vi "uTTA_Write_UCF_File.vi"(4 "TC_Channels":T1(array[cluster]), 6 "TSP_Channels":T1(array[cluster]), 8 "error in (no error)":errorcluster, 10 "Inputs":T2 {"I_Sense Offset" format="%#3.3pA"; "I_Sense Gain" format="%#3.3pA/Digit"; "CH_I Offset" format="%#3.3pA"; "CH_I Gain" format="%#3.3pA/Digit"; "CH0 PA3 Offset" format="%#3.3pV"; "CH0 PA3 Gain" format="%#3.3pV/Digit"; "CH0 PA2 Offset" format="%#3.3pV"; "CH0 PA2 Gain" format="%#3.3pV/Digit"; "CH0 PA1 Offset" format="%#3.3pV"; "CH0 PA1 Gain" format="%#3.3pV/Digit"; "CH0 PA0 Offset" format="%#3.3pV"; "CH0 PA0 Gain" format="%#3.3pV/Digit"; "CH3 PA0 Offset" format="%#3.3pV"; "CH3 PA0 Gain" format="%#3.3pV/Digit"; "CH2 PA0 Offset" format="%#3.3pV"; "CH2 PA0 Gain" format="%#3.3pV/Digit"; "CH1 PA0 Offset" format="%#3.3pV"; "CH1 PA0 Gain" format="%#3.3pV/Digit"; "Voffs1 Offset" format="%#3.3pV"; "Voffs1 Gain" format="%#3.3pV/Digit"; "Voffs0 Offset" format="%#3.3pV"; "CH3 Diff Gain" format="%#3.3pV/V"; "CH2 Diff Gain" format="%#3.3pV/V"; "CH1 Diff Gain" format="%#3.3pV/V"; "Voffs0 Gain" format="%#3.3pV/Digit"; "CH0 Diff Gain" format="%#3.3pV/V"}, 11 "selected path":path) -> (0 "error out":errorcluster, 3 "file path":path)   [LabVIEW 2021]
uses:
  CTL_uTTA_BlockDiagCal.ctl
  <vilib>/Utility/config.llb/NI_LVConfig.lvlib
panel:
  # "G0"
  # "G1"
  # "G2"
  # "G3"
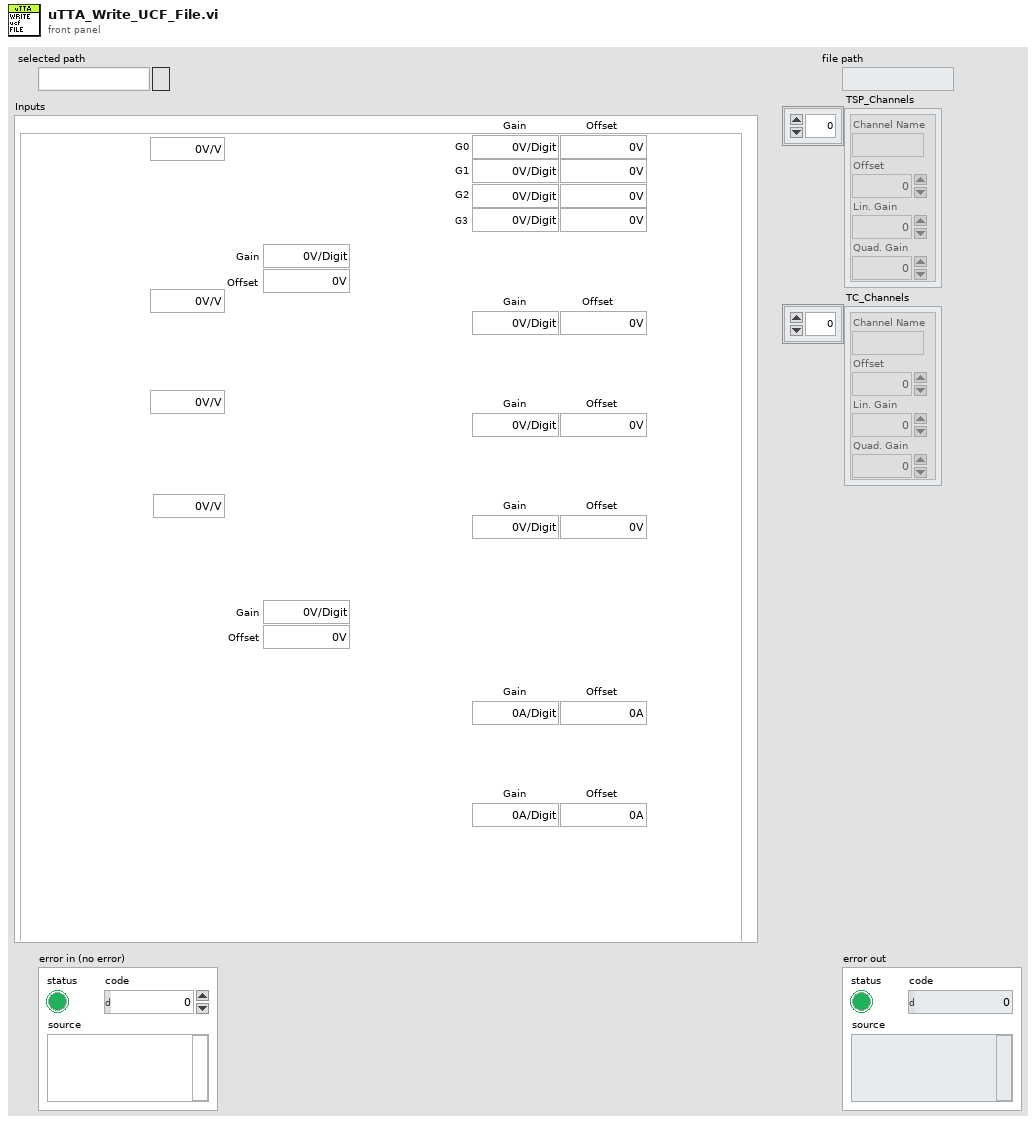
[diagram p1: front panel]
types:
  T1 = cluster{"Channel Name":string, "Offset":dbl, "Lin. Gain":dbl, "Quad. Gain":dbl}[]
  T2 = typedef "CTL_uTTA_BlockDiagCal.ctl" = cluster{"CH0 Diff Gain":dbl, "Voffs0 Gain":dbl, "CH1 Diff Gain":dbl, "CH2 Diff Gain":dbl, "CH3 Diff Gain":dbl, "Voffs0 Offset":dbl, "Voffs1 Gain":dbl, "Voffs1 Offset":dbl, "CH1 PA0 Gain":dbl, "CH1 PA0 Offset":dbl, "CH2 PA0 Gain":dbl, "CH2 PA0 Offset":dbl, "CH3 PA0 Gain":dbl, "CH3 PA0 Offset":dbl, "CH0 PA0 Gain":dbl, "CH0 PA0 Offset":dbl, "CH0 PA1 Gain":dbl, "CH0 PA1 Offset":dbl, "CH0 PA2 Gain":dbl, "CH0 PA2 Offset":dbl, "CH0 PA3 Gain":dbl, "CH0 PA3 Offset":dbl, "CH_I Gain":dbl, "CH_I Offset":dbl, "I_Sense Gain":dbl, "I_Sense Offset":dbl}
  T3 = typedef "NI_LVConfig.lvlib/Config Data RefNum.ctl" = refnum<k1>
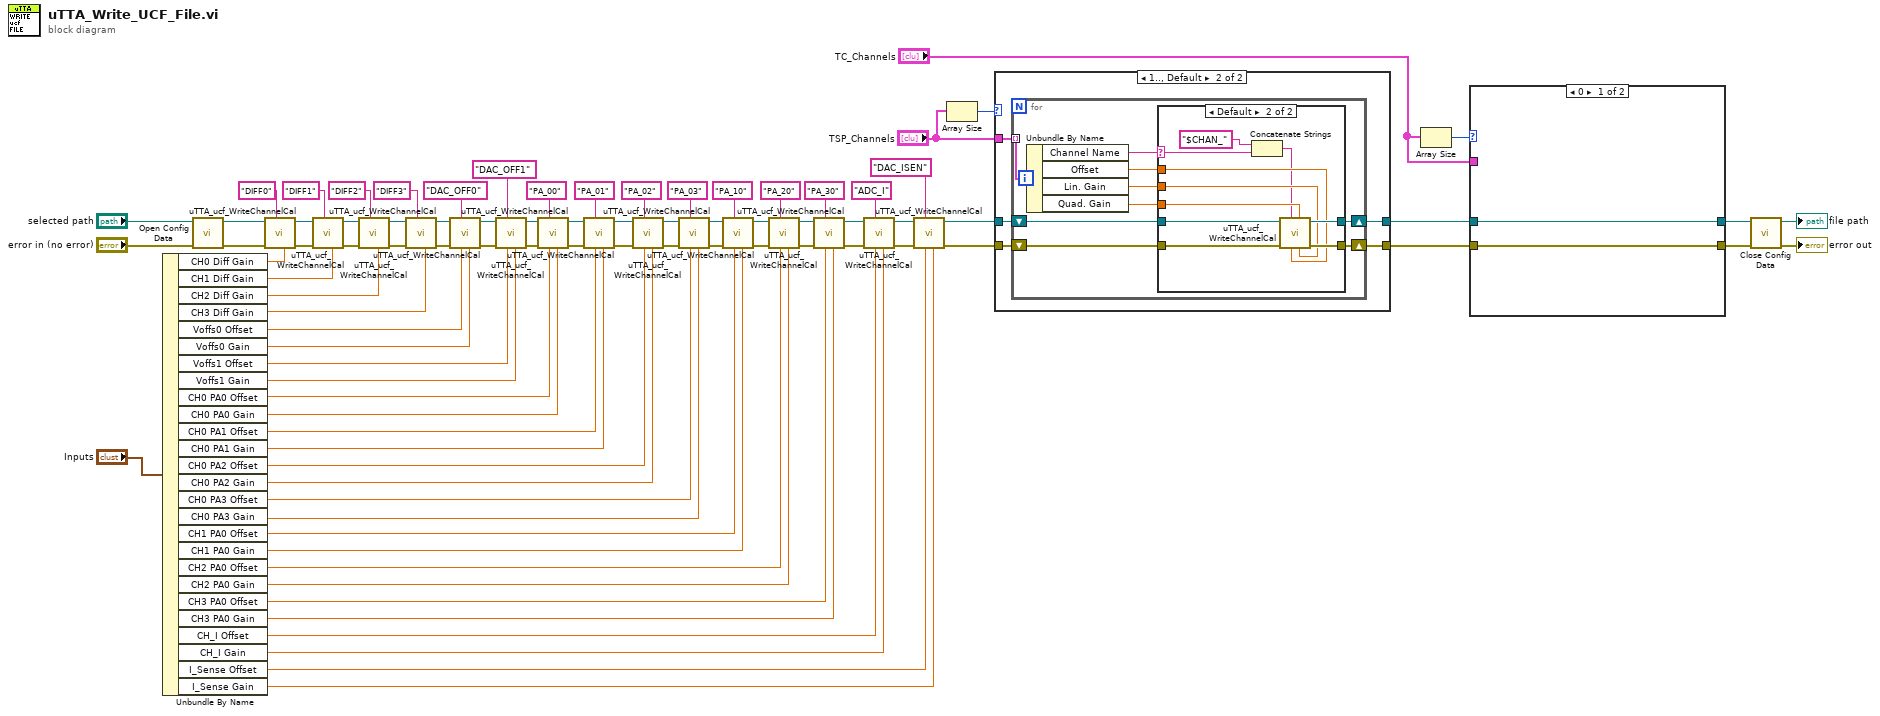
[diagram p0: block diagram]
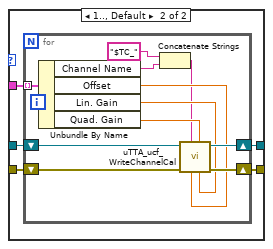
[diagram p2: hidden frame]
diagram:
  n1 = Unbundle By Name("Inputs") -> ("CH0 Diff Gain"=w28:dbl, "CH1 Diff Gain"=w29:dbl, "CH2 Diff Gain"=w30:dbl, "CH3 Diff Gain"=w33:dbl, "Voffs0 Offset"=w36:dbl, "Voffs0 Gain"=w37:dbl, "Voffs1 Offset"=w46:dbl, "Voffs1 Gain"=w47:dbl, "CH0 PA0 Offset"=w48:dbl, "CH0 PA0 Gain"=w49:dbl, "CH0 PA1 Offset"=w50:dbl, "CH0 PA1 Gain"=w51:dbl, "CH0 PA2 Offset"=w52:dbl, "CH0 PA2 Gain"=w53:dbl, "CH0 PA3 Offset"=w60:dbl, "CH0 PA3 Gain"=w61:dbl, "CH1 PA0 Offset"=w62:dbl, "CH1 PA0 Gain"=w63:dbl, "CH2 PA0 Offset"=w64:dbl, "CH2 PA0 Gain"=w65:dbl, "CH3 PA0 Offset"=w68:dbl, "CH3 PA0 Gain"=w69:dbl, "CH_I Offset"=w75:dbl, "CH_I Gain"=w76:dbl, "I_Sense Offset"=w15:dbl, "I_Sense Gain"=w14:dbl)
  n2 = call <vilib>:"Open Config Data.vi"("error in (no error)"="error in (no error)", "configuration file path"="selected path") -> ("error out"=w18:errorcluster, "refnum"=w19:T3)  [unwired: 7 in, 1 out]
  n3 = call "uTTA_ucf_WriteChannelCal.vi"("LinGain"=w28, "Section"="DIFF0" ("section"), "error in (no error)"=w18, "ucf FileRef in"=w19) -> ("error out"=w24:errorcluster, "ucf FileRef out"=w25:T3)  [unwired: 6 in]
  n4 = call "uTTA_ucf_WriteChannelCal.vi"("LinGain"=w29, "Section"="DIFF1" ("section"), "error in (no error)"=w24, "ucf FileRef in"=w25) -> ("error out"=w26:errorcluster, "ucf FileRef out"=w27:T3)  [unwired: 6 in]
  n5 = call "uTTA_ucf_WriteChannelCal.vi"("LinGain"=w30, "Section"="DIFF2" ("section"), "error in (no error)"=w26, "ucf FileRef in"=w27) -> ("error out"=w31:errorcluster, "ucf FileRef out"=w32:T3)  [unwired: 6 in]
  n6 = call "uTTA_ucf_WriteChannelCal.vi"("LinGain"=w33, "Section"="DIFF3" ("section"), "error in (no error)"=w31, "ucf FileRef in"=w32) -> ("error out"=w34:errorcluster, "ucf FileRef out"=w35:T3)  [unwired: 6 in]
  n7 = call "uTTA_ucf_WriteChannelCal.vi"("LinGain"=w37, "Offset"=w36, "Section"="DAC_OFF0", "error in (no error)"=w34, "ucf FileRef in"=w35) -> ("error out"=w38:errorcluster, "ucf FileRef out"=w39:T3)  [unwired: 5 in]
  n8 = call "uTTA_ucf_WriteChannelCal.vi"("LinGain"=w47, "Offset"=w46, "Section"="DAC_OFF1", "error in (no error)"=w38, "ucf FileRef in"=w39) -> ("error out"=w40:errorcluster, "ucf FileRef out"=w41:T3)  [unwired: 5 in]
  n9 = call "uTTA_ucf_WriteChannelCal.vi"("LinGain"=w49, "Offset"=w48, "Section"="PA_00", "error in (no error)"=w40, "ucf FileRef in"=w41) -> ("error out"=w42:errorcluster, "ucf FileRef out"=w43:T3)  [unwired: 5 in]
  n10 = call "uTTA_ucf_WriteChannelCal.vi"("LinGain"=w51, "Offset"=w50, "Section"="PA_01", "error in (no error)"=w42, "ucf FileRef in"=w43) -> ("error out"=w44:errorcluster, "ucf FileRef out"=w45:T3)  [unwired: 5 in]
  n11 = call "uTTA_ucf_WriteChannelCal.vi"("LinGain"=w53, "Offset"=w52, "Section"="PA_02", "error in (no error)"=w44, "ucf FileRef in"=w45) -> ("error out"=w54:errorcluster, "ucf FileRef out"=w55:T3)  [unwired: 5 in]
  n12 = call "uTTA_ucf_WriteChannelCal.vi"("LinGain"=w61, "Offset"=w60, "Section"="PA_03", "error in (no error)"=w54, "ucf FileRef in"=w55) -> ("error out"=w56:errorcluster, "ucf FileRef out"=w57:T3)  [unwired: 5 in]
  n13 = call "uTTA_ucf_WriteChannelCal.vi"("LinGain"=w63, "Offset"=w62, "Section"="PA_10", "error in (no error)"=w56, "ucf FileRef in"=w57) -> ("error out"=w58:errorcluster, "ucf FileRef out"=w59:T3)  [unwired: 5 in]
  n14 = call "uTTA_ucf_WriteChannelCal.vi"("LinGain"=w65, "Offset"=w64, "Section"="PA_20", "error in (no error)"=w58, "ucf FileRef in"=w59) -> ("error out"=w66:errorcluster, "ucf FileRef out"=w67:T3)  [unwired: 5 in]
  n15 = call "uTTA_ucf_WriteChannelCal.vi"("LinGain"=w69, "Offset"=w68, "Section"="PA_30", "error in (no error)"=w66, "ucf FileRef in"=w67) -> ("error out"=w73:errorcluster, "ucf FileRef out"=w74:T3)  [unwired: 5 in]
  n16 = call "uTTA_ucf_WriteChannelCal.vi"("LinGain"=w76, "Offset"=w75, "Section"="ADC_I", "error in (no error)"=w73, "ucf FileRef in"=w74) -> ("error out"=w17:errorcluster, "ucf FileRef out"=w16:T3)  [unwired: 5 in]
  n17 = call "uTTA_ucf_WriteChannelCal.vi"("LinGain"=w14, "Offset"=w15, "Section"="DAC_ISEN", "error in (no error)"=w17, "ucf FileRef in"=w16) -> ("error out"=w11:errorcluster, "ucf FileRef out"=w12:T3)  [unwired: 5 in]
  n18 = Array Size(array="TSP_Channels") -> (size(s)=w3:i32)
  n19 = case shown="1.., Default" w3 {
    tunnel: w12 -> [w88 w93]
    tunnel: w11 -> [w87 w92]
    tunnel: [w88 w91] -> w8
    tunnel: [w87 w90] -> w7
    tunnel: "TSP_Channels" -> [_ w89]
    frame 0 {
    }
    frame 1.., Default {
      n20 = for {
        shift-right: [w99] -> w91
        shift-left: w93 -> [w101]
        shift-right: [w98] -> w90
        shift-left: w92 -> [w100]
        tunnel: w89 -> [w102] mode=indexing
        n21 = Unbundle By Name(w102) -> ("Channel Name"=w94:string, "Offset"=w95:dbl, "Lin. Gain"=w96:dbl, "Quad. Gain"=w97:dbl)
        n22 = case shown="Default" w94 {
          selector: w94 -> [_ w105]
          tunnel: w101 -> [w104 w114]
          tunnel: w100 -> [w103 w113]
          tunnel: [w104 w112] -> w99
          tunnel: [w103 w111] -> w98
          tunnel: w97 -> [_ w110]
          tunnel: w96 -> [_ w109]
          tunnel: w95 -> [_ w108]
          frame "OFF" {
          }
          frame Default {
            n23 = Concatenate Strings("$CHAN_" ("string"), w105) -> (w106:string)
            n24 = call "uTTA_ucf_WriteChannelCal.vi"("LinGain"=w109, "QuadGain"=w110, "Offset"=w108, "Section"=w106, "error in (no error)"=w113, "ucf FileRef in"=w114) -> ("error out"=w111:errorcluster, "ucf FileRef out"=w112:T3)  [unwired: 4 in]
          }
        }
      }
    }
  }
  n25 = Array Size(array="TC_Channels") -> (size(s)=w1:i32)
  n26 = case shown="0" w1 {
    tunnel: w8 -> [w116 w121]
    tunnel: w7 -> [w115 w120]
    tunnel: [w116 w119] -> w6
    tunnel: [w115 w118] -> w5
    tunnel: "TC_Channels" -> [_ w117]
    frame 0 {
    }
    frame 1.., Default {
      n27 = for {
        shift-right: [w129] -> w119
        shift-left: w121 -> [w131]
        shift-right: [w128] -> w118
        shift-left: w120 -> [w130]
        tunnel: w117 -> [w132] mode=indexing
        n28 = Unbundle By Name(w132) -> ("Channel Name"=w123:string, "Offset"=w125:dbl, "Lin. Gain"=w126:dbl, "Quad. Gain"=w127:dbl)
        n29 = Concatenate Strings("$TC_" ("string"), w123) -> (w122:string)
        n30 = call "uTTA_ucf_WriteChannelCal.vi"("LinGain"=w126, "QuadGain"=w127, "Offset"=w125, "Section"=w122, "error in (no error)"=w130, "ucf FileRef in"=w131) -> ("error out"=w128:errorcluster, "ucf FileRef out"=w129:T3)  [unwired: 4 in]
      }
    }
  }
  n31 = call <vilib>:"Close Config Data.vi"("error in (no error)"=w5, "refnum"=w6) -> ("error out"=→"error out":errorcluster, "file path"=→"file path":path)  [unwired: 8 in]
